vi "Host sender&receiver.vi"() -> ()   [LabVIEW 2017]
panel:
  out "Received String from myRIO":string
  in  "stop":bool
  out "Sent Number to myRIO":string
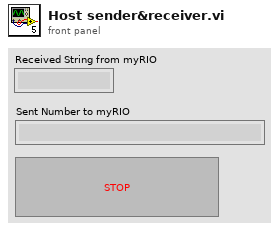
[diagram p1: front panel]
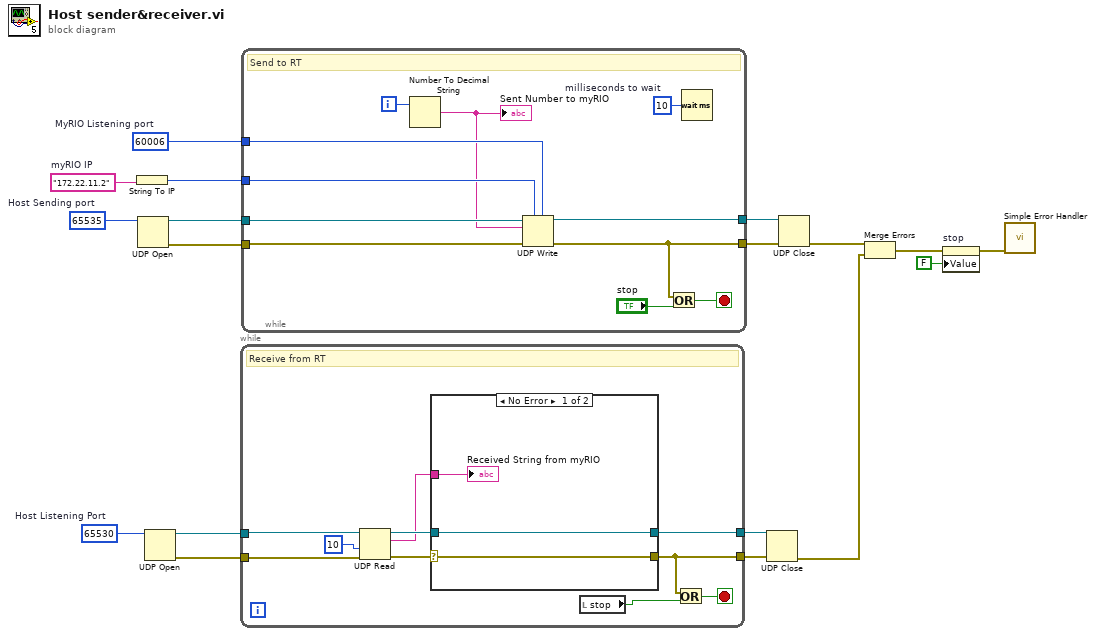
[diagram p0: block diagram]
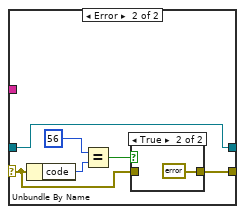
[diagram p2: hidden frame]
diagram:
  w8 = u16 65530  # Host Listening Port
  w13 = u16 60006  # MyRIO Listening port
  w15 = "172.22.11.2"  # myRIO IP
  w18 = u16 65535  # Host Sending port
  n1 = String To IP(1:w15) -> (0:w14:u32)
  n2 = UDP Open(11:w18) -> (port=w16:refnum<k16>, 0:w17:errorcluster)  [unwired: 4 in, 1 out]
  n3 = UDP Open(11:w8) -> (port=w10:refnum<k16>, 0:w9:errorcluster)  [unwired: 4 in, 1 out]
  n4 = while {
    tunnel: w10 -> [w28]
    tunnel: w9 -> [w27]
    tunnel: [w20] -> w7
    tunnel: [w22] -> w6
    stop <- w21 stop-if-true
    # "Receive from RT"
    n5 = UDP Read(connection ID=w28, timeout ms (25000)=10, 8:w27) -> (data out=w23:string, error out=w25:errorcluster, 3:w24:refnum<k16>)  [unwired: 1 in, 2 out]
    n6 = case shown="No Error" w25 {
      selector: w25 -> [w31 w33]
      tunnel: w24 -> [w30 w32]
      tunnel: w23 -> [w29 _]
      tunnel: [w31 w34] -> w20
      tunnel: [w30 w32] -> w22
      frame No Error {
        "Received String from myRIO" <- w29
      }
      frame Error {
        n7 = Unbundle By Name(w33) -> ("code"=w37:i32)
        n8 = Equal?(x=56, y=w37) -> (x = y?=w35:bool)
        n9 = case shown="True" w35 {
          tunnel: [w38 errorcluster {"status"=FALSE, "code"=0, "source"=""} ("error constant")] -> w34
          tunnel: w33 -> [w38 _]
          frame False {
          }
          frame True {
          }
        }
      }
    }
    n10 = local read "stop"() -> (w19:bool)
    n11 = Or(x=w20, y=w19) -> (x .or. y?=w21:bool)
  }
  n12 = while {
    tunnel: w17 -> [w48]
    tunnel: w16 -> [w49]
    tunnel: w14 -> [w47]
    tunnel: w13 -> [w46]
    tunnel: [w43] -> w12
    tunnel: [w41] -> w11
    i -> [w45]
    stop <- w42 stop-if-true
    w50 = u32 10  # milliseconds to wait
    # "Send to RT"
    n13 = Number To Decimal String(number=w45) -> (decimal integer string=w44:string)  [unwired: 1 in]
    "Sent Number to myRIO" <- w44
    n14 = UDP Write(address=w47, port or service name=w46, connection ID=w49, data in=w44, 8:w48) -> (error out=w41:errorcluster, 3:w43:refnum<k16>)  [unwired: 1 in]
    n15 = Or(x=w41, y="stop") -> (x .or. y?=w42:bool)
    n16 = Wait (ms)(milliseconds to wait=w50) -> ()  [unwired: 1 out]
  }
  n17 = UDP Close(connection ID=w6, 8:w7) -> (error out=w4:errorcluster)  [unwired: 1 out]
  n18 = UDP Close(connection ID=w12, 8:w11) -> (error out=w5:errorcluster)  [unwired: 1 out]
  n19 = Merge Errors(w5, w4) -> (w3:errorcluster)
  n20 = property on="stop" class="Bool (strict)"(error in=w3, "Value"=FALSE ("stop")) -> (error out=w2:errorcluster)  [unwired: 1 in, 1 out]
  n21 = call <vilib>:"Simple Error Handler.vi"("error in (no error)"=w2) -> ()  [unwired: 4 in, 5 out]
